vi "Enum_To_Text.vi"(9 "Parameter":T1) -> (1 "Text":string)   [LabVIEW 2019]
uses:
  (C2K_ADC)_Parameter.ctl
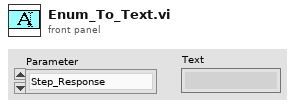
[diagram p1: front panel]
types:
  T1 = typedef "(C2K_ADC)_Parameter.ctl" = enum16{"Step_Response"}
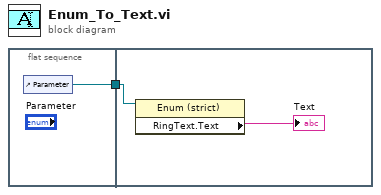
[diagram p0: block diagram]
diagram:
  n1 = flat-sequence {
    tunnel: [w2] -> w1
    tunnel: w1 -> [w3]
    frame #0 {
      n2 = control-ref of="Parameter"() -> (w2:refnum<vi>)
    }
    frame #1 {
      n3 = property class="Enum (strict)"(reference=w3) -> ("RingText.Text"=→"Text":string)  [unwired: 1 in, 2 out]
    }
  }
